vi "calc_approach_coords.vi"(8 "manip transform":T1={"theta (deg)"=0.0, "X sc factor (px/step)"=1.0, "Y sc factor (px/step)"=1.0, "zero loc (x,y,z)"=[0.0, 0.0], "flip y?"=FALSE, "flip x?"=FALSE, "gamma (deg)"=25.0, "flip z?"=FALSE, "Z sc factor (px/step)"=0.1098, "actuator"={"Actuator COM"="COM3", "Actuator type"=enum."Scientifica"}, "safe space (steps)"=[-69533, 0, -29190]} {"Y sc factor (px/step)" format="%#_13g"; "X sc factor (px/step)" format="%#_13g"; "theta (deg)" format="%#_13g"}, 10 "Z_topP":dbl, 11 "cell location (steps, pipette coord system)":dbl[](array[numeric])) -> (0 "distToDescend":i32, 3 "(x,y,z)_pP_TOPOFSLICE":i32[](array[numeric]))   [LabVIEW 2015]
uses:
  pipette cleaning/pressure box/cleaning_soft/controls/actuator_type.ctl
  pipette cleaning/pressure box/cleaning_soft/controls/actuator_cluster.ctl
  transform_properties_actuators.ctl
panel:
  out "Y_pP":dbl
  out "X_pP":dbl
  # "top of slice"
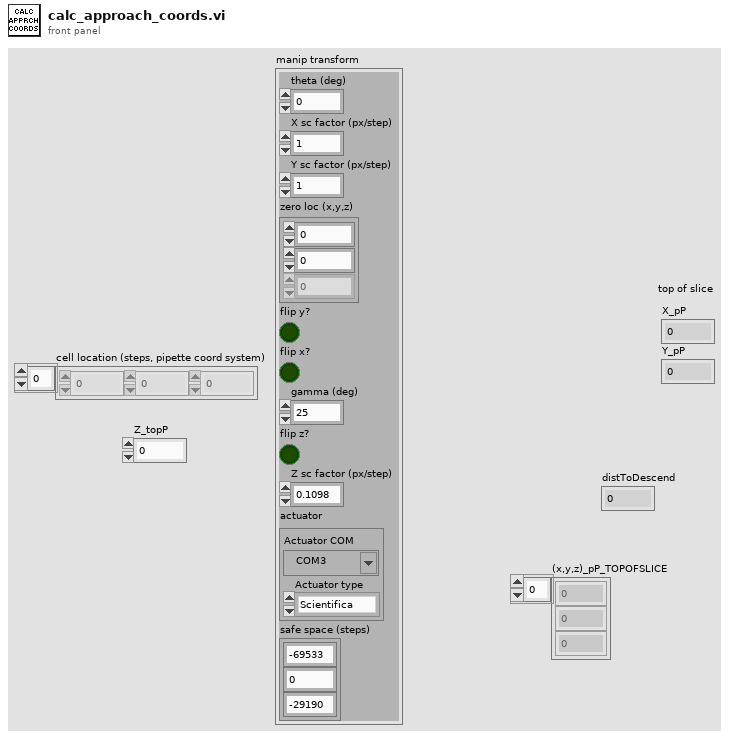
[diagram p1: front panel]
types:
  T1 = typedef "transform_properties_actuators.ctl" = cluster{"theta (deg)":dbl, "X sc factor (px/step)":dbl, "Y sc factor (px/step)":dbl, "zero loc (x,y,z)":dbl[], "flip y?":bool, "flip x?":bool, "gamma (deg)":dbl, "flip z?":bool, "Z sc factor (px/step)":dbl, "actuator":T2, "safe space (steps)":i32[]}
  T2 = typedef "actuator_cluster.ctl" = cluster{"Actuator COM":refnum<visa-resource-name>, "Actuator type":T3}
  T3 = typedef "actuator_type.ctl" = enum16{"Scientifica", "Sutter", "Demo", "Off"}
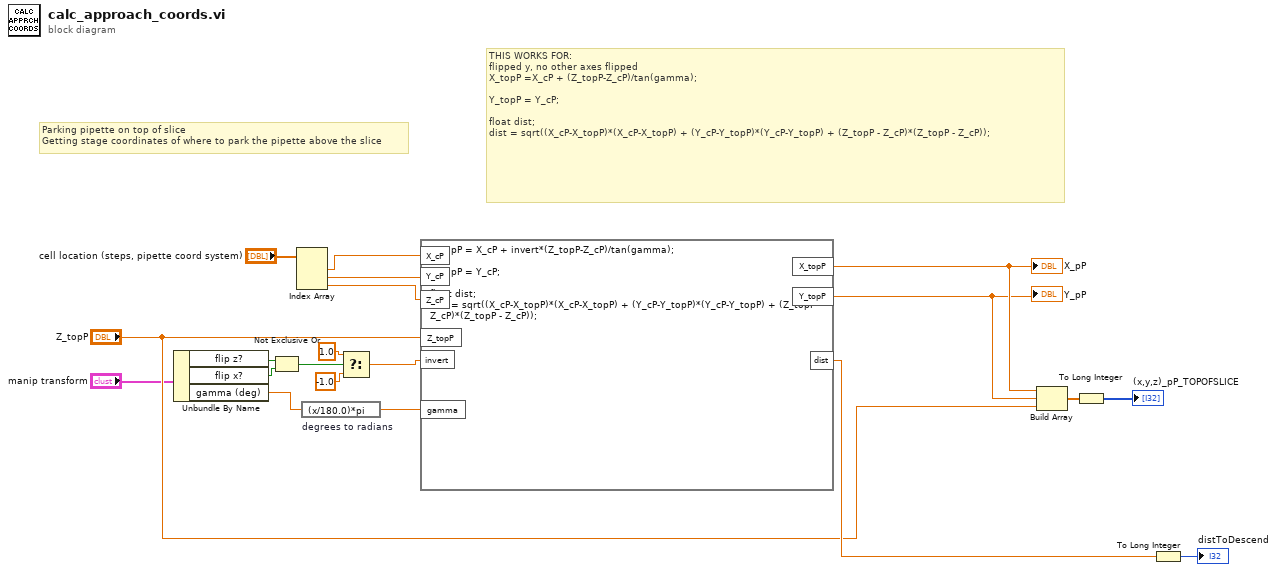
[diagram p0: block diagram]
diagram:
  # "THIS WORKS FOR:\nflipped y, no other axes flipped\nX_topP =X_cP + (Z_topP-Z_cP)/tan(gamma);\n\nY_topP = Y_cP;\n\nfloat dist;\ndist = sqrt((X_cP-X_topP)*(X_cP-X_topP) + (Y_cP-Y_topP)*(Y_cP-Y_topP) + (Z_topP - Z_cP)*(Z_topP - Z_cP));"
  # "Parking pipette on top of slice\nGetting stage coordinates of where to park the pipette above the slice"
  n1 = Unbundle By Name("manip transform") -> ("flip z?"=w2:bool, "flip x?"=w3:bool, "gamma (deg)"=w7:dbl)
  n2 = Not Exclusive Or(1:w3, 2:w2) -> (0:w1:bool)
  n3 = Index Array(array="cell location (steps, pipette coord system)") -> (element #1=w13:dbl, element #2=w12:dbl, element #3=w11:dbl)  [unwired: 3 in]
  n4 = expression code="(x/180.0)*pi" "degrees to radians"(w7) -> (w20:dbl)
  n5 = Select(t=1.0, s=w1, f=-1.0) -> (s? t:f=w4:dbl)
  n6 = formula code="X_topP = X_cP + invert*(Z_topP-Z_cP)/tan(gamma);\n\nY_topP = Y_cP;\n\nfloat dist;\ndist = sqrt((X_cP-X_topP)*(X_cP-X_topP) + (Y_cP-Y_topP)*(Y_cP-Y_topP) + (Z_topP - Z_cP)*(Z_topP - Z_cP));"("X_cP"=w13, "Y_cP"=w12, "Z_cP"=w11, "Z_topP"="Z_topP", "gamma"=w20, "invert"=w4) -> ("X_topP"=w16:dbl, "Y_topP"=w15:dbl, "dist"=w10:dbl)
  "X_pP" <- w16
  "Y_pP" <- w15
  n7 = Build Array(w16, w15, "Z_topP") -> (w19:dbl[])
  n8 = To Long Integer(number=w19) -> (32bit integer=→"(x,y,z)_pP_TOPOFSLICE":i32[])
  n9 = To Long Integer(number=w10) -> (32bit integer=→"distToDescend":i32)
